vi "Filter Test Cases.vi"(8 "error in (no error)":errorcluster, 11 "Classes to Filter":path[](array[path])) -> (0 "error out":errorcluster, 3 "Filtered Classes":path[](array[path]))   [LabVIEW 2020, in "Test Finder.lvclass"]
uses:
  Test Finder.lvclass
  LUnit Test Case.lvclass
  Test Finder.lvclass/Test Finder.ctl
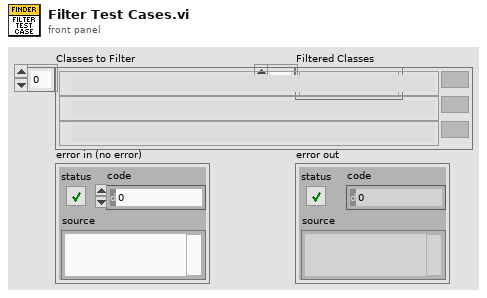
[diagram p1: front panel]
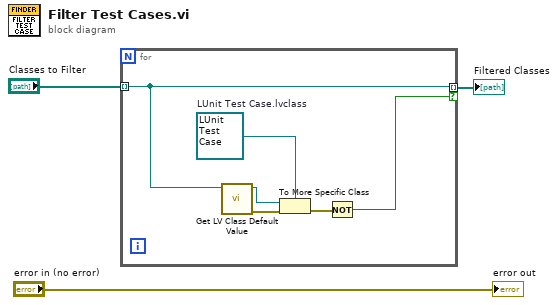
[diagram p0: block diagram]
diagram:
  n1 = for {
    tunnel: "Classes to Filter" -> [w4] mode=indexing
    tunnel: [w4] -> w2 mode=indexing if=w5
    w7 = refnum<class "LUnit Test Case.lvclass"> refnum  # LUnit Test Case.lvclass
    n2 = call <vilib>:"Get LV Class Default Value.vi"("class path"=w4) -> ("error out"=w9:errorcluster, "object"=w8:refnum<class>)  [unwired: 9 in]
    n3 = To More Specific Class(target class=w7, reference=w8, error in=w9) -> (error out=w6:errorcluster)  [unwired: 1 out]
    n4 = Not(x=w6) -> (.not. x?=w5:bool)
  }
  "Filtered Classes" <- w2
  "error out" <- "error in (no error)"
